vi "Get_Argument.vi"(1 "Argument":string, 2 "Argument List":string[](array[string])) -> (0 "Enabled":bool)   [LabVIEW 2011]
doc: "This VI is a simple macro that examines the supplied argument list (a string array) and tries to locate a match corresponding to the contents of the \"Argument\" parameter. In the growth sequence editor code, the value of a boolean argument is determined only by its existance in the \"Argument List\"."
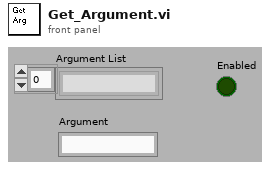
[diagram p1: front panel]
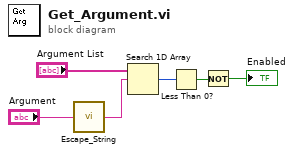
[diagram p0: block diagram]
diagram:
  n1 = call "Escape_String.vi"("Input String"="Argument") -> ("Escaped String"=w1:string)
  n2 = Search 1D Array(1D array="Argument List", element=w1) -> (index of element=w5:i32)  [unwired: 1 out]
  n3 = Less Than 0?(x=w5) -> (x < 0?=w4:bool)
  n4 = Not(x=w4) -> (.not. x?=→"Enabled":bool)
